vi "waitForNewResults.vi"(7 "address":string, 8 "error in (no error)":errorcluster, 11 "Instrument.Lockin in":refnum<class "Instrument.Lockin.lvclass">) -> (0 "error out":errorcluster, 2 "Results":dbl[][](array[numeric]), 3 "Instrument.Lockin out":refnum<class "Instrument.Lockin.lvclass">)   [LabVIEW 2016]
uses:
  Instrument.Lockin/Instrument.Lockin.lvclass
panel:
  in  "Port":u16
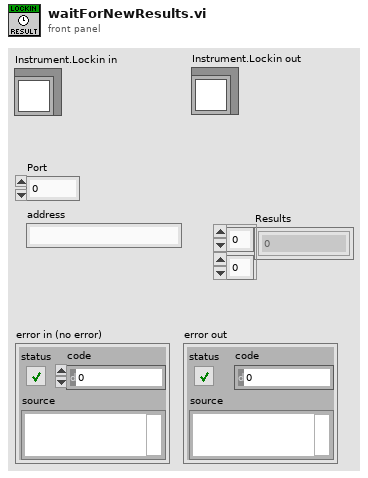
[diagram p1: front panel]
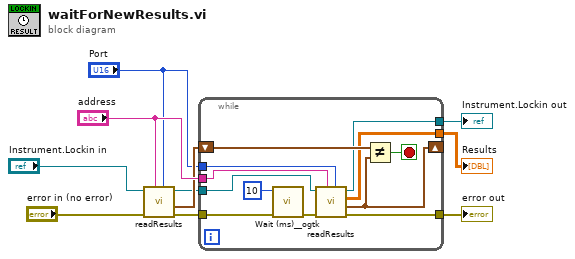
[diagram p0: block diagram]
diagram:
  n1 = call "readResults.vi"("Port"="Port", "address"="address", "error in (no error)"="error in (no error)", "Instrument.Lockin in"="Instrument.Lockin in") -> ("error out"=w8:errorcluster, "Time Stamp"=w5:timestamp, "Instrument.Lockin out"=w3:refnum<class "Instrument.Lockin.lvclass">)  [unwired: 4 in, 1 out]
  n2 = while {
    shift-right: [w15] -> _
    shift-left: w5 -> [w20]
    tunnel: w8 -> [w21]
    tunnel: [w17] -> w10
    tunnel: "address" -> [w16]
    tunnel: [w14] -> w6
    tunnel: w3 -> [w13]
    tunnel: [w12] -> w2
    tunnel: "Port" -> [w11]
    stop <- w22 stop-if-true
    n3 = call <userlib>:"Wait (ms)__ogtk.vi"("error in (no error)"=w21, "milliseconds to wait"=u32 10) -> ("error out"=w18:errorcluster)  [unwired: 8 in, 1 out]
    n4 = call "readResults.vi"("Port"=w11, "address"=w16, "error in (no error)"=w18, "Instrument.Lockin in"=w13) -> ("error out"=w17:errorcluster, "Time Stamp"=w15:timestamp, "Results"=w14:dbl[][], "Instrument.Lockin out"=w12:refnum<class "Instrument.Lockin.lvclass">)  [unwired: 4 in]
    n5 = Not Equal?(x=w20, y=w15) -> (x != y?=w22:bool)
  }
  "error out" <- w10
  "Results" <- w6
  "Instrument.Lockin out" <- w2
